vi "Read.vi"(8 "error in (no error)":errorcluster, 10 "Data Ref":T1, 11 "VeriStand DSF in":refnum<class "VeriStand DSF.Framework.lvclass">) -> (0 "error out":errorcluster, 3 "VeriStand DSF out":refnum<class "VeriStand DSF.Framework.lvclass">)   [LabVIEW 2017, in "Data Sharing Framework Engine.lvlib" / "VeriStand DSF.Framework.lvclass"]
uses:
  VeriStand DSF.Framework.lvclass
  C:/github/data-sharing-framework/Data Sharing Framework/Builds/Current/Data Sharing Framework Core/Data Sharing Framework Core.lvlibp/Engine/Framework/Framework.lvclass
  <vilib>/NI Veristand/Custom Device API/Data Table Ref.ctl
  Builds/Current/Data Sharing Framework Core/Data Sharing Framework Core.lvlibp/Engine/Framework/Framework.lvclass
  <vilib>/NI VeriStand/Custom Device API/Custom Device API.lvlib
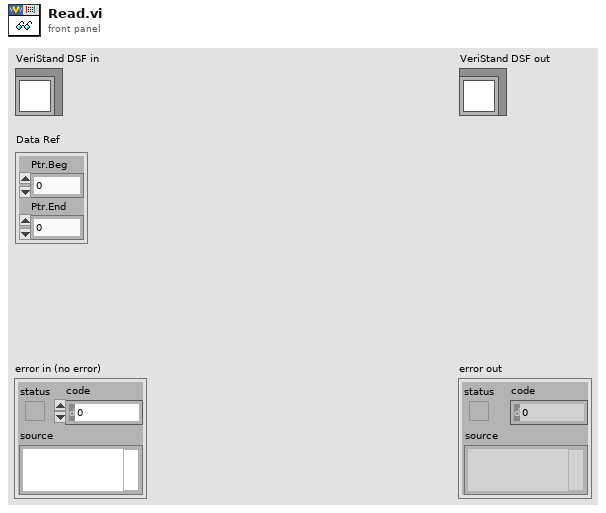
[diagram p1: front panel]
types:
  T1 = typedef "Custom Device API.lvlib/Data Table Ref.ctl" = cluster{"Ptr.Beg":u64, "Ptr.End":u64}
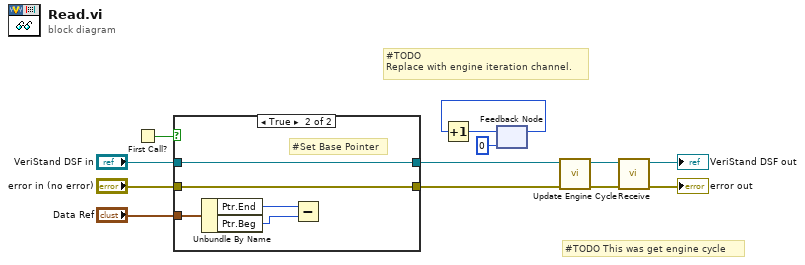
[diagram p0: block diagram]
diagram:
  # "#TODO This was get engine cycle"
  # "#TODO\nReplace with engine iteration channel."
  n1 = First Call?() -> (First Call?: T/F=w7:bool)
  n2 = case shown="True" w7 {
    tunnel: "VeriStand DSF in" -> [w15 w18]
    tunnel: "error in (no error)" -> [w14 w17]
    tunnel: [w15 w18] -> w4
    tunnel: [w14 w17] -> w2
    tunnel: "Data Ref" -> [_ w20]
    frame False {
    }
    frame True {
      # "#Set Base Pointer"
      n3 = Unbundle By Name(w20) -> ("Ptr.End"=w19:u64, "Ptr.Beg"=w16:u64)
      n4 = Subtract(x=w19, y=w16) -> ()  [unwired: 1 out]
    }
  }
  n5 = feedback #1(u64 0 ("iteration")) -> (w3:u64)
  n6 = Increment(x=w3) -> (x+1=w8:u64)
  n7 = feedback-in #1(w8) -> ()
  n8 = call-dynamic "Update Engine Cycle.vi"("error in (no error)"=w2, "Framework in"=w4) -> ("error out"=w11:errorcluster, "Framework out"=w13:refnum<class "VeriStand DSF.Framework.lvclass">)  [unwired: 8 in]
  n9 = call "Receive.vi"("error in (no error)"=w11, "Framework in"=w13) -> ("error out"=→"error out":errorcluster, "Framework out"=→"VeriStand DSF out":refnum<class "VeriStand DSF.Framework.lvclass">)  [unwired: 8 in]
